vi "Create destination paths.vi"() -> ()   [LabVIEW 2015]
uses:
  Create destinations/Files state.ctl
  <vilib>/Utility/sysdir.llb/System Directory Type.ctl
  <vilib>/Utility/config.llb/Read Key (Boolean).vi
  <vilib>/Utility/config.llb/Write Key (Boolean).vi
  <vilib>/Utility/config.llb/Write Key (Path).vi
  <vilib>/Utility/config.llb/NI_LVConfig.lvlib
panel:
  out "Tab Control":enum32{"Message", "Next"}(tab)
  in  "Skip":bool
  in  "Continue":bool
  # "First time setup\n\nWe're setting up the files and folders required to store data about the newspapers on your system. This ensures that your data is never sent to anyone, not even us. You'll be able to export it should you need to. Please wait for us to finish, this should only take a few moments."
  # "Add in your newspapers\n\nWe've finished setting up the files and folders required to function. Click Continue to add or edit the data about the newspapers you subscribe to, or click Skip to skip this step.\n\nIf you're installing Newspaper Bill Calculator for the first time, it is recommended to proceed."
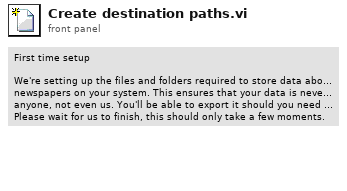
[diagram p1: front panel]
types:
  T1 = typedef "Files state.ctl" = enum16{"Init", "Open INI", "Store to INI", "Create files", "Edit papers", "Exit"}
  T2 = typedef "System Directory Type.ctl" = i32
  T3 = typedef "NI_LVConfig.lvlib/Config Data RefNum.ctl" = refnum<k1>
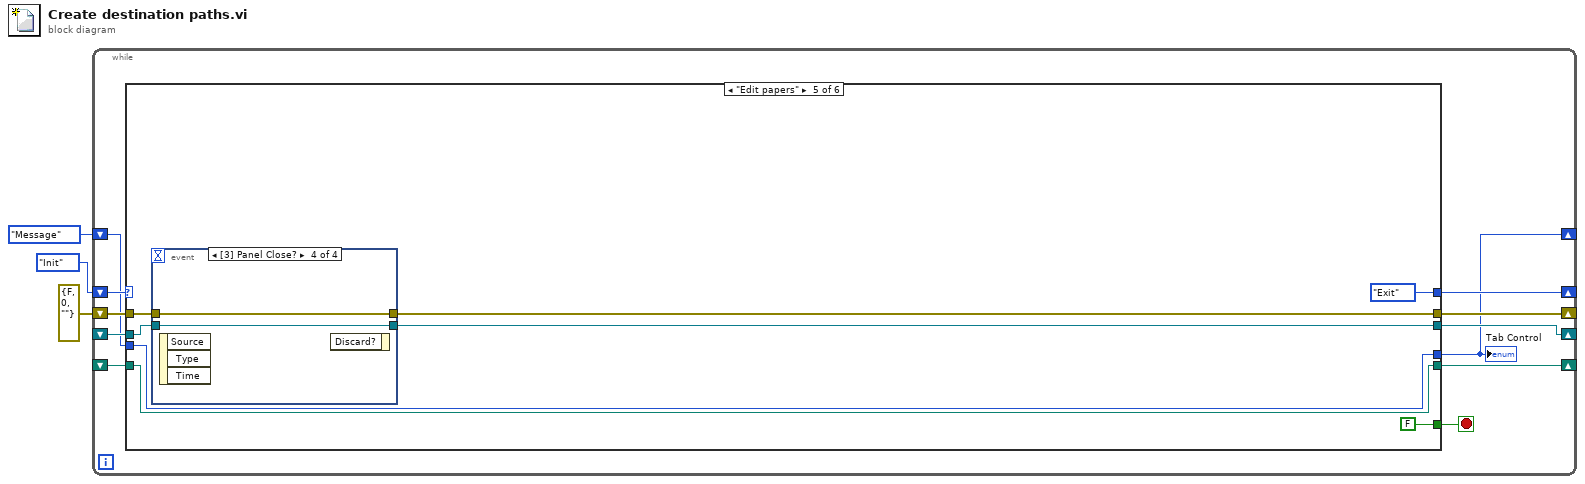
[diagram p0: block diagram]
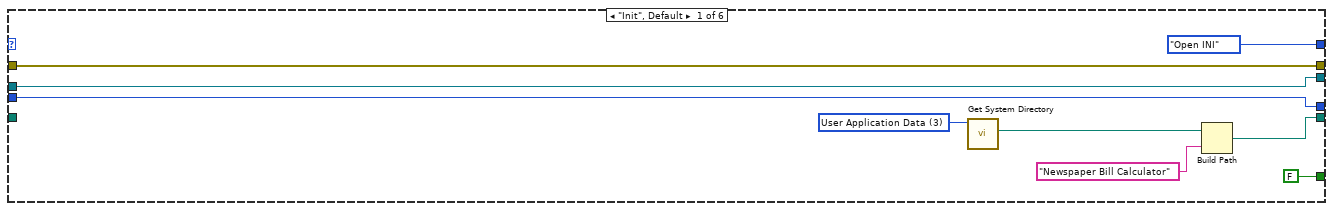
[diagram p2: hidden frame]
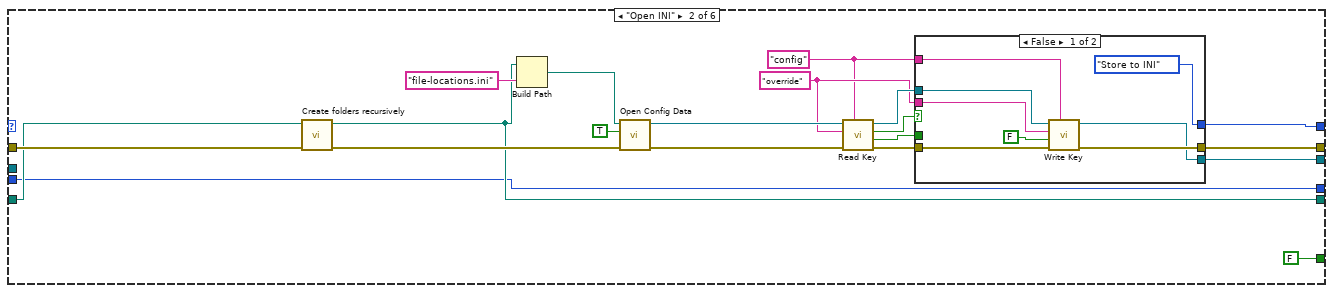
[diagram p3: hidden frame]
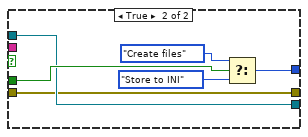
[diagram p4: hidden frame]
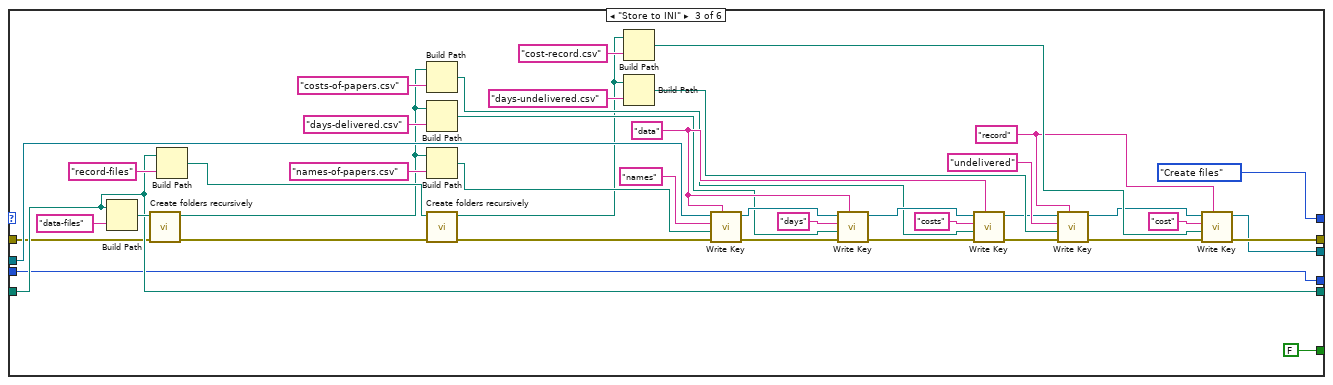
[diagram p5: hidden frame]
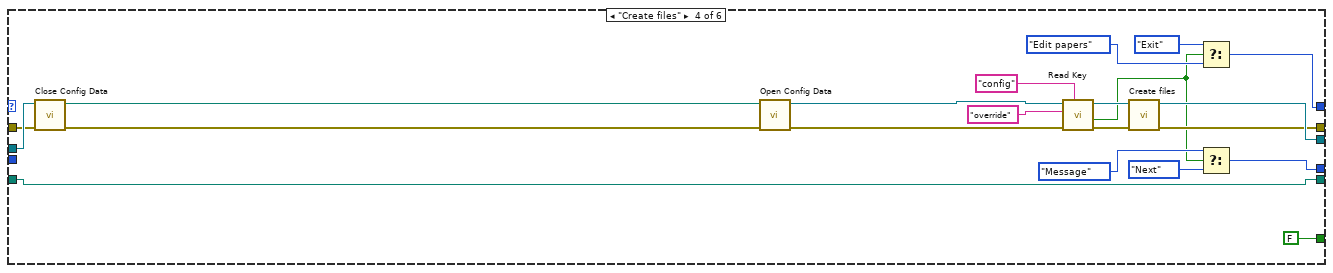
[diagram p6: hidden frame]
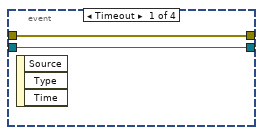
[diagram p7: hidden frame]
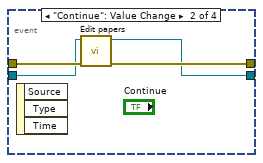
[diagram p8: hidden frame]
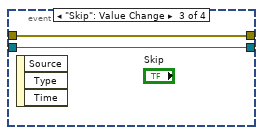
[diagram p9: hidden frame]
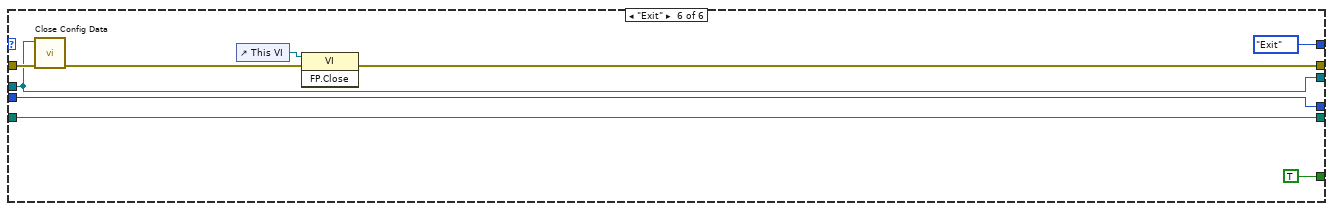
[diagram p10: hidden frame]
diagram:
  n1 = while {
    shift-right: [w13] -> _
    shift-left: Files_state."Init" -> [w14]
    shift-right: [w11] -> _
    shift-left: errorcluster {"status"=FALSE, "code"=0, "source"=""} ("error out") -> [w12]
    shift-right: [w10] -> _
    shift-left: _ -> [w9]
    shift-right: [w6] -> _
    shift-left: _ -> [w7]
    shift-right: [w5] -> _
    shift-left: enum32{"Message", "Next"}."Message" ("Tab Control 2") -> [w4]
    stop <- w8 stop-if-true
    n2 = case shown="\"Edit papers\"" w14 {
      tunnel: [Files_state."Open INI" w36 Files_state."Create files" w107 Files_state."Exit" Files_state."Exit"] -> w13
      tunnel: w12 -> [w17 w27 w61 w118 w121 w142]
      tunnel: [w17 w31 w78 w115 w122 w139] -> w11
      tunnel: [w22 w30 w77 w116 w123 w141] -> w10
      tunnel: w9 -> [w22 _ w92 w119 w120 w141]
      tunnel: [FALSE FALSE FALSE FALSE FALSE TRUE] -> w8
      tunnel: w7 -> [_ w26 w65 w100 w127 w146]
      tunnel: [w16 w25 w65 w100 w127 w146] -> w6
      tunnel: [w15 w24 w58 w102 w124 w143] -> w5
      tunnel: w4 -> [w15 w24 w58 _ w124 w143]
      frame "Init", Default {
        w19 = T2 3 items=["User Home"=0, "User Desktop"=1, "User Documents"=2, "User Application Data"=3, "User Preferences"=4, "User Temporary"=5, "Public Documents"=6, "Public Application Data"=7, "Public Preferences"=8, "Public Cache"=13, "System Core Libraries"=9, "System Installed Libraries"=10, "Application Files"=11, "Boot Volume Root"=12] ("system directory type")
        n3 = call <vilib>:"Get System Directory.vi"("system directory type"=w19) -> ("system directory"=w20:path)  [unwired: 10 in]
        n4 = Build Path(base path=w20, name or relative path="Newspaper Bill Calculator") -> (appended path=w16:path)
      }
      frame "Open INI" {
        w33 = "override" ("key")
        w32 = "config" ("section")
        n5 = call "Create folders recursively.vi"("error in (no error)"=w27, "Path in"=w26) -> ("error out"=w28:errorcluster, "Path out"=w25:path)  [unwired: 8 in]
        n6 = Build Path(base path=w25, name or relative path="file-locations.ini") -> (appended path=w42:path)
        n7 = call <vilib>:"Open Config Data.vi"("error in (no error)"=w28, "create file if necessary (T)"=TRUE, "configuration file path"=w42) -> ("error out"=w38:errorcluster, "refnum"=w39:T3)  [unwired: 6 in, 1 out]
        n8 = call-poly <vilib>:"Read Key.vi"("section"=w32, "error in (no error)"=w38, "key"=w33, "refnum"=w39) -> ("error out"=w34:errorcluster, "value"=w29:bool, "found?"=w37:bool, "refnum out"=w35:T3)  [unwired: 4 in]
        n9 = case shown="False" w37 {
          tunnel: [Files_state."Store to INI" w54] -> w36
          tunnel: w35 -> [w50 w53]
          tunnel: w34 -> [w49 w52]
          tunnel: w33 -> [w48 _]
          tunnel: w32 -> [w47 _]
          tunnel: [w45 w52] -> w31
          tunnel: [w44 w53] -> w30
          tunnel: w29 -> [_ w55]
          frame False {
            n10 = call-poly <vilib>:"Write Key.vi"("section"=w47, "error in (no error)"=w49, "value"=FALSE, "key"=w48, "refnum"=w50) -> ("error out"=w45:errorcluster, "refnum out"=w44:T3)  [unwired: 4 in, 1 out]
          }
          frame True {
            n11 = Select(t=Files_state."Create files", s=w55, f=Files_state."Store to INI") -> (s? t:f=w54:T1)
          }
        }
      }
      frame "Store to INI" {
        w79 = "record" ("section")
        w84 = "data" ("section")
        n12 = Build Path(base path=w65, name or relative path="data-files") -> (appended path=w93:path)
        n13 = call "Create folders recursively.vi"("error in (no error)"=w61, "Path in"=w93) -> ("error out"=w60:errorcluster, "Path out"=w63:path)  [unwired: 8 in]
        n14 = Build Path(base path=w65, name or relative path="record-files") -> (appended path=w71:path)
        n15 = Build Path(base path=w63, name or relative path="costs-of-papers.csv") -> (appended path=w81:path)
        n16 = Build Path(base path=w63, name or relative path="days-delivered.csv") -> (appended path=w82:path)
        n17 = Build Path(base path=w63, name or relative path="names-of-papers.csv") -> (appended path=w91:path)
        n18 = call "Create folders recursively.vi"("error in (no error)"=w60, "Path in"=w71) -> ("error out"=w59:errorcluster, "Path out"=w62:path)  [unwired: 8 in]
        n19 = Build Path(base path=w62, name or relative path="cost-record.csv") -> (appended path=w80:path)
        n20 = Build Path(base path=w62, name or relative path="days-undelivered.csv") -> (appended path=w72:path)
        n21 = call-poly <vilib>:"Write Key.vi"("section"=w84, "error in (no error)"=w59, "value"=w91, "key"="names", "refnum"=w92) -> ("error out"=w88:errorcluster, "refnum out"=w87:T3)  [unwired: 4 in, 1 out]
        n22 = call-poly <vilib>:"Write Key.vi"("section"=w84, "error in (no error)"=w88, "value"=w82, "key"="days", "refnum"=w87) -> ("error out"=w85:errorcluster, "refnum out"=w86:T3)  [unwired: 4 in, 1 out]
        n23 = call-poly <vilib>:"Write Key.vi"("section"=w84, "error in (no error)"=w85, "value"=w81, "key"="costs", "refnum"=w86) -> ("error out"=w66:errorcluster, "refnum out"=w67:T3)  [unwired: 4 in, 1 out]
        n24 = call-poly <vilib>:"Write Key.vi"("section"=w79, "error in (no error)"=w66, "value"=w72, "key"="undelivered", "refnum"=w67) -> ("error out"=w75:errorcluster, "refnum out"=w76:T3)  [unwired: 4 in, 1 out]
        n25 = call-poly <vilib>:"Write Key.vi"("section"=w79, "error in (no error)"=w75, "value"=w80, "key"="cost", "refnum"=w76) -> ("error out"=w78:errorcluster, "refnum out"=w77:T3)  [unwired: 4 in, 1 out]
      }
      frame "Create files" {
        n26 = call <vilib>:"Close Config Data.vi"("error in (no error)"=w118, "refnum"=w119) -> ("error out"=w99:errorcluster, "file path"=w117:path)  [unwired: 8 in]
        n27 = call <vilib>:"Open Config Data.vi"("error in (no error)"=w99, "configuration file path"=w117) -> ("error out"=w112:errorcluster, "refnum"=w113:T3)  [unwired: 7 in, 1 out]
        n28 = call-poly <vilib>:"Read Key.vi"("section"="config", "error in (no error)"=w112, "key"="override", "refnum"=w113) -> ("error out"=w109:errorcluster, "value"=w101:bool, "refnum out"=w108:T3)  [unwired: 4 in, 1 out]
        n29 = call "Create files.vi"("error in (no error)"=w109, "INI Refnum in"=w108) -> ("error out"=w115:errorcluster, "INI Refnum out"=w116:T3)  [unwired: 8 in]
        n30 = Select(t=Files_state."Exit", s=w101, f=Files_state."Edit papers") -> (s? t:f=w107:T1)
        n31 = Select(t=enum32{"Message", "Next"}."Message" ("Tab Control 2"), s=w101, f=enum32{"Message", "Next"}."Next" ("Tab Control 2")) -> (s? t:f=w102:enum32{"Message", "Next"})
      }
      frame "Edit papers" {
        n32 = event shown="[3] Panel Close?" {
          selector: _ -> [_ _ _ _]
          dyn-events: _ -> [_ _ _ _]
          timeout: _ -> [_ _ _ _]
          tunnel: w121 -> [w129 w133 w134 w136]
          tunnel: [w129 w132 w134 w136] -> w122
          tunnel: w120 -> [w128 w131 w135 w137]
          tunnel: [w128 w130 w135 w137] -> w123
          event Timeout {
            n33 = event-data() -> ()  [unwired: 1 in, 3 out]
          }
          event "Continue": Value Change {
            n34 = event-data() -> ()  [unwired: 1 in, 3 out]
            n35 = call "Edit papers.vi"("Error In"=w133, "INI refnum in"=w131) -> ("Error Out"=w132:errorcluster, "INI refnum Out"=w130:T3)  [unwired: 8 in]
          }
          event "Skip": Value Change {
            n36 = event-data() -> ()  [unwired: 1 in, 3 out]
          }
          event Panel Close? {
            n37 = event-data() -> ()  [unwired: 1 in, 3 out]
            n38 = event-data() -> ()  [unwired: 2 in, 1 out]
          }
        }
      }
      frame "Exit" {
        n39 = call <vilib>:"Close Config Data.vi"("error in (no error)"=w142, "refnum"=w141) -> ("error out"=w138:errorcluster)  [unwired: 8 in, 1 out]
        n40 = control-ref of="This VI"() -> (w140:refnum<vi>)
        n41 = invoke class="VI" method="FP.Close"(reference=w140, error in=w138) -> (error out=w139:errorcluster)  [unwired: 1 in, 2 out]
      }
    }
    "Tab Control" <- w5
  }
